vi "FlatToRichmeasurement_DataPoint.vi"(5 "OutputClusterType":T1, 11 "InputCluster":T2) -> (3 "OutputCluster":T1)   [LabVIEW 2021, in "Measurement_server.lvlib"]
uses:
  Measurement_server.lvlib
  measurement_DataPoint_Flat.ctl
  measurement_DataPoint.ctl
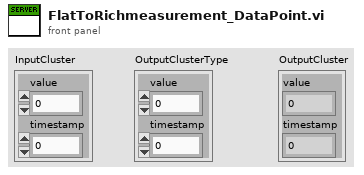
[diagram p1: front panel]
types:
  T1 = typedef "Measurement_server.lvlib/measurement_DataPoint.ctl" = cluster{"value":dbl, "timestamp":i64}
  T2 = typedef "Measurement_server.lvlib/measurement_DataPoint_Flat.ctl" = cluster{"value":dbl, "timestamp":i64}
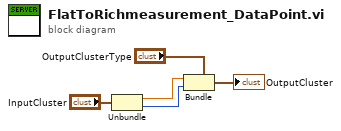
[diagram p0: block diagram]
diagram:
  n1 = Unbundle "Unbundle"("InputCluster") -> ("value"=w2:dbl, "timestamp"=w1:i64)
  n2 = Bundle "Bundle"(cluster="OutputClusterType", "value"=w2, "timestamp"=w1) -> (→"OutputCluster":T1)
